vi "Arrays With Enums - No Type Defs.vi"(8 "Array Of Clusters With Enums 2":T1(array[cluster])=[{"Numeric"=11.0, "Inner Cluster - Level 1"={"String"="Number 11", "Boolean"=TRUE, "Enum"=enum."BBB", "Numbers Enum"=enum."Four", "Text & Picture Control"=1, "Array"=[{"Numeric"=22.0, "String"="Number 22", "Text Ring"=111.0, "Array Of Enums"=[enum."One", enum."Five", enum."Three", enum."Four"], "Text Ring Control"=3.0}, {"Numeric"=111.0, "String"="Number 111", "Text Ring"=7788.0, "Array Of Enums"=[enum."Zero", enum."One", enum."Two", enum."Three"], "Text Ring Control"=5.0}]}}, {"Numeric"=5.0, "Inner Cluster - Level 1"={"String"="FooBAR", "Boolean"=TRUE, "Enum"=enum."EEEE", "Numbers Enum"=enum."Five", "Text & Picture Control"=5, "Array"=[{"Numeric"=78945.0, "String"="Numeric Value 78945", "Text Ring"=5566.0, "Array Of Enums"=[enum."Five", enum."Four", enum."Three", enum."Two"], "Text Ring Control"=2.0}, {"Numeric"=1122.0, "String"="aaaaaa", "Text Ring"=4455.0, "Array Of Enums"=[enum."Two", enum."One", enum."Zero"], "Text Ring Control"=4.0}]}}] {"Inner Cluster - Level 1"."Text & Picture Control" items=["Home Sweet Home!", "Another Piece Of The Puzzle", "Hmmm ????", "The Connector Pane", "Look At The Fish", "Its A Turtle!"]; "Inner Cluster - Level 1"."Array"."Text Ring Control" items=["Text Value 0", "Text Value 1", "Text Value 2", "Text Value 3", "Text Value 5", "Text Value 6"]; "Inner Cluster - Level 1"."Array"."Text Ring" items=["Text Ring Value 1"=111, "Text Ring Value 2"=2233, "Text Ring Value 3"=4455, "Text Ring Value 4"=5566, "Text Ring Value 5"=7788]}, 9 "Array Of Clusters With Enums":T2(array[cluster])=[{"Numeric"=11.0, "Inner Cluster - Level 1"={"String"="ABCDE", "Boolean"=TRUE, "Enum"=enum."EEEE", "Numbers Enum"=enum."Two", "Cluster"={"Numeric"=11.0, "String"="FGHIJ", "Text Ring"=5566}, "Array Of Text Rings"=[1, 4]}}, {"Numeric"=8899.0, "Inner Cluster - Level 1"={"String"="Numeric Value 8899", "Boolean"=FALSE, "Enum"=enum."AAA", "Numbers Enum"=enum."Five", "Cluster"={"Numeric"=45.0, "String"="Numeric Value 45", "Text Ring"=111}, "Array Of Text Rings"=[4, 4]}}] {"Inner Cluster - Level 1"."Array Of Text Rings" items=["Text Value 0", "Text Value 1", "Text Value 2", "Text Value 3", "Text Value 5", "Text Value 6"]; "Inner Cluster - Level 1"."Cluster"."Text Ring" items=["Text Ring Value 1"=111, "Text Ring Value 2"=2233, "Text Ring Value 3"=4455, "Text Ring Value 4"=5566, "Text Ring Value 5"=7788]}, 10 "Array Of Text Ring":i32[](array[ring])=[1, 3, 4] items=["Text Value 0", "Text Value 1", "Text Value 2", "Text Value 3", "Text Value 5", "Text Value 6"], 11 "Array Of Enums":T3(array[ring])=[enum."One", enum."Three", enum."Zero", enum."Four"]) -> ()   [LabVIEW 2012]
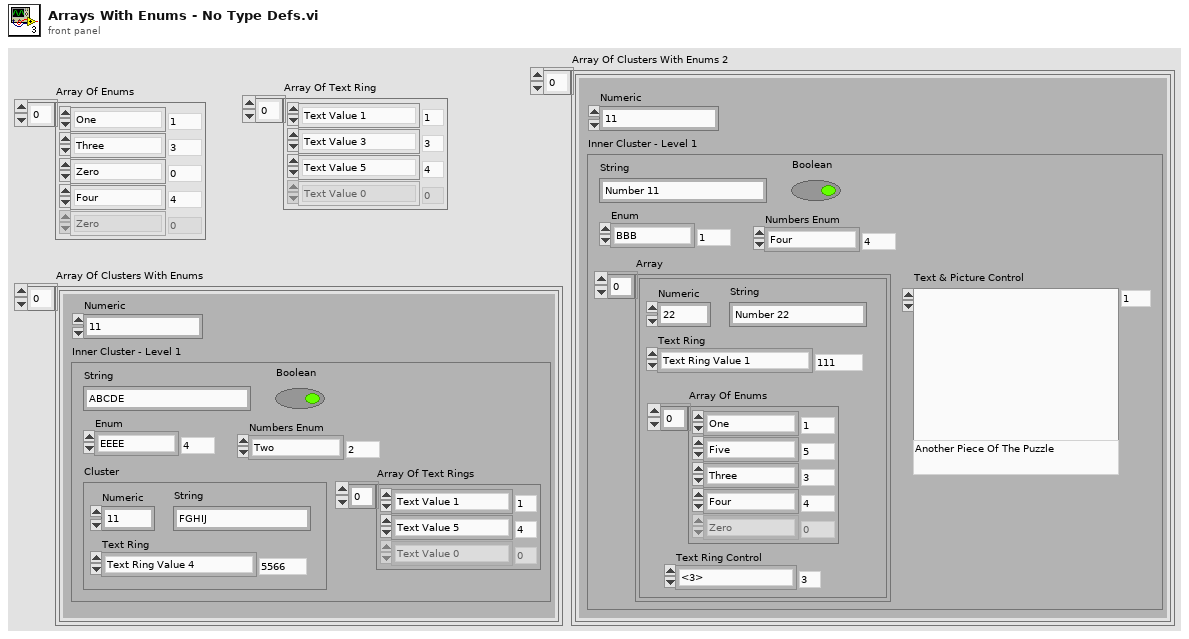
[diagram p1: front panel]
types:
  T1 = cluster{"Numeric":dbl, "Inner Cluster - Level 1":cluster{"String":string, "Boolean":bool, "Enum":enum32{"AAA", "BBB", "CCCC", "DDDD", "EEEE"}, "Numbers Enum":enum16{"Zero", "One", "Two", "Three", "Four", "Five"}, "Text & Picture Control":i32, "Array":cluster{"Numeric":dbl, "String":string, "Text Ring":sgl, "Array Of Enums":enum16{"Zero", "One", "Two", "Three", "Four", "Five"}[], "Text Ring Control":dbl}[]}}[]
  T2 = cluster{"Numeric":dbl, "Inner Cluster - Level 1":cluster{"String":string, "Boolean":bool, "Enum":enum16{"AAA", "BBB", "CCCC", "DDDD", "EEEE"}, "Numbers Enum":enum16{"Zero", "One", "Two", "Three", "Four", "Five"}, "Cluster":cluster{"Numeric":dbl, "String":string, "Text Ring":i32}, "Array Of Text Rings":i16[]}}[]
  T3 = enum32{"Zero", "One", "Two", "Three", "Four", "Five"}[]
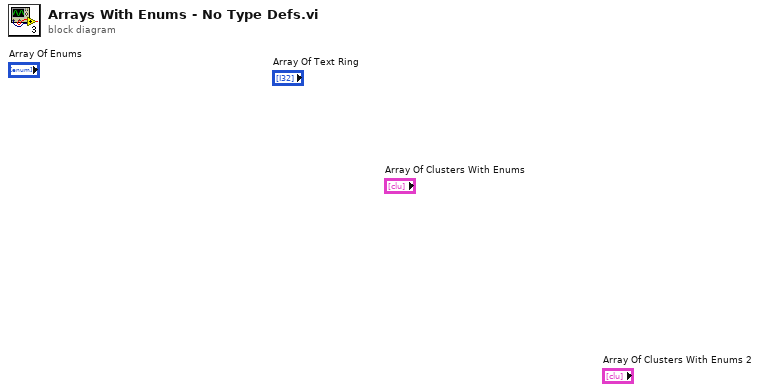
[diagram p0: block diagram]
diagram:
